vi "Run_Core.vi"(0 "Message Popup in":refnum<class "SMU.lvclass">, 11 "error in (no error)":errorcluster) -> (4 "Message Popup out":refnum<class "SMU.lvclass">, 6 "Return":variant, 15 "error out":errorcluster)   [LabVIEW 2016, in "SMU.lvclass"]
uses:
  SMU.lvclass
  SMU.lvclass/SMU.ctl
  <instrlib>/niDCPower/nidcpower.llb/niDCPower Measurement Type.ctl
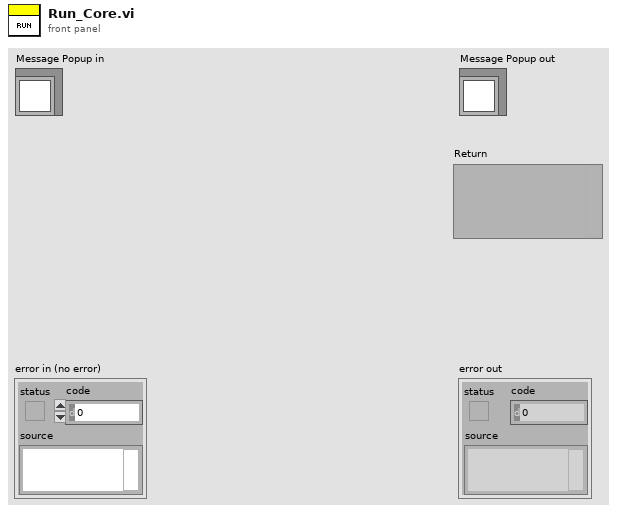
[diagram p1: front panel]
types:
  T1 = typedef "SMU.lvclass/Function List.ctl" = enum16{"init", "source voltage", "source current", "measure voltage", "close", "close all"}
  T2 = typedef "niDCPower Measurement Type.ctl" = i32
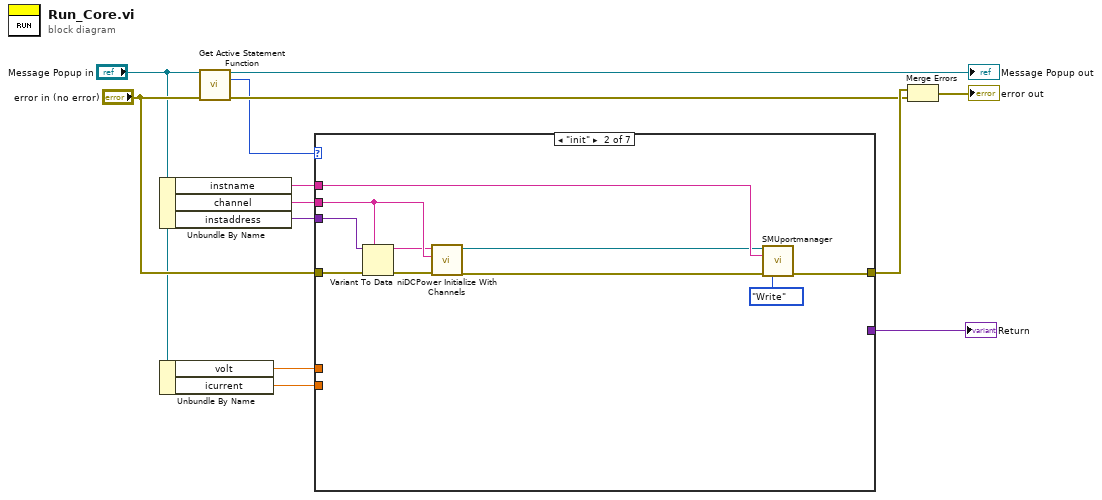
[diagram p0: block diagram]
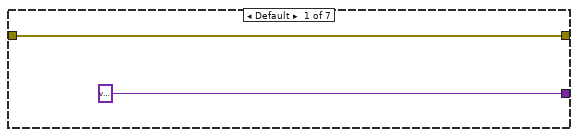
[diagram p2: hidden frame]
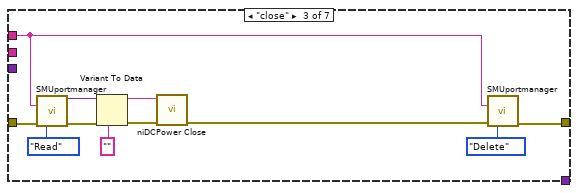
[diagram p3: hidden frame]
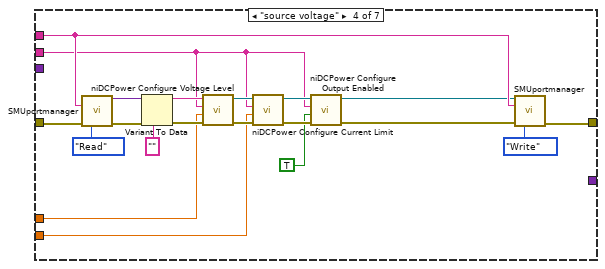
[diagram p4: hidden frame]
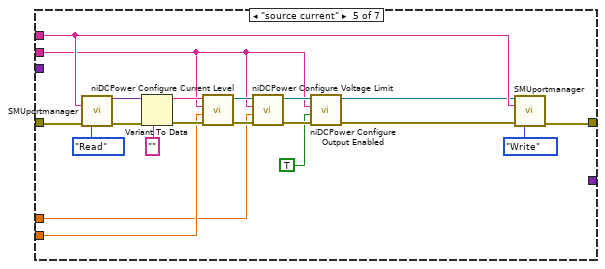
[diagram p5: hidden frame]
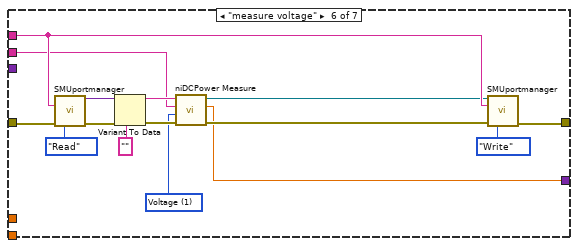
[diagram p6: hidden frame]
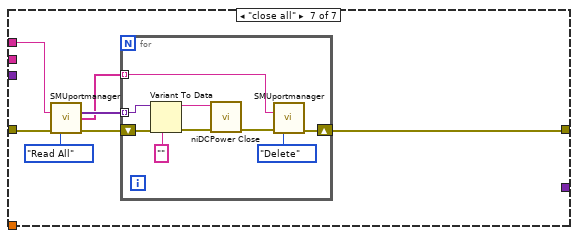
[diagram p7: hidden frame]
diagram:
  n1 = Unbundle By Name("Message Popup in") -> ("instname"=w5:string, "channel"=w4:string, "instaddress"=w11:variant)
  n2 = Unbundle By Name("Message Popup in") -> ("volt"=w2:dbl, "icurrent"=w1:dbl)
  n3 = call "Get Active Statement Function.vi"("Statement in"="Message Popup in", "error in (no error)"="error in (no error)") -> ("Statement out"=→"Message Popup out":refnum<class "SMU.lvclass">, "Function List"=w7:T1, "error out"=w9:errorcluster)  [unwired: 11 in]
  n4 = case shown="\"init\"" w7 {
    tunnel: "error in (no error)" -> [w15 w24 w28 w51 w71 w86 w95]
    tunnel: w11 -> [_ w25 _ _ _ _ _]
    tunnel: [w15 w19 w34 w54 w74 w89 w98] -> w10
    tunnel: [variant ("lefttocomma") _ _ _ _ w77 _] -> w6
    tunnel: w5 -> [_ w22 w27 w50 w70 w85 w94]
    tunnel: w4 -> [_ w17 _ w39 w61 w79 _]
    tunnel: w2 -> [_ _ _ w45 w57 _ _]
    tunnel: w1 -> [_ _ _ w43 w58 _ _]
    frame Default {
    }
    frame "init" {
      n5 = Variant To Data(error in=w24, type=w17, Variant=w25) -> (data=w16:string, error out=w23:errorcluster)
      n6 = call <instrlib>:"niDCPower Initialize With Channels.vi"("error in (no error)"=w23, "channels"=w17, "resource name"=w16) -> ("error out"=w21:errorcluster, "instrument handle out"=w20:refnum<k15>)  [unwired: 7 in]
      n7 = call "SMUportmanager.vi"("port in"=w20, "Name"=w22, "error in (no error)"=w21, "Action"=enum16{"Read", "Write", "Read All", "Delete"}."Write") -> ("error out"=w19:errorcluster)  [unwired: 8 in, 3 out]
    }
    frame "close" {
      n8 = call "SMUportmanager.vi"("Name"=w27, "error in (no error)"=w28, "Action"=enum16{"Read", "Write", "Read All", "Delete"}."Read") -> ("port"=w26:variant, "error out"=w30:errorcluster)  [unwired: 9 in, 2 out]
      n9 = Variant To Data(error in=w30, type="", Variant=w26) -> (data=w33:string, error out=w32:errorcluster)
      n10 = call <instrlib>:"niDCPower Close.vi"("error in (no error)"=w32, "instrument handle"=w33) -> ("error out"=w31:errorcluster)  [unwired: 9 in]
      n11 = call "SMUportmanager.vi"("Name"=w27, "error in (no error)"=w31, "Action"=enum16{"Read", "Write", "Read All", "Delete"}."Delete") -> ("error out"=w34:errorcluster)  [unwired: 9 in, 3 out]
    }
    frame "source voltage" {
      n12 = call "SMUportmanager.vi"("Name"=w50, "error in (no error)"=w51, "Action"=enum16{"Read", "Write", "Read All", "Delete"}."Read") -> ("port"=w49:variant, "error out"=w53:errorcluster)  [unwired: 9 in, 2 out]
      n13 = Variant To Data(error in=w53, type="", Variant=w49) -> (data=w46:string, error out=w48:errorcluster)
      n14 = call <instrlib>:"niDCPower Configure Voltage Level.vi"("error in (no error)"=w48, "voltage level"=w45, "channel name"=w39, "instrument handle"=w46) -> ("error out"=w47:errorcluster, "instrument handle out"=w44:refnum<k15>)  [unwired: 6 in]
      n15 = call <instrlib>:"niDCPower Configure Current Limit.vi"("error in (no error)"=w47, "current limit"=w43, "channel name"=w39, "instrument handle"=w44) -> ("error out"=w41:errorcluster, "instrument handle out"=w42:refnum<k15>)  [unwired: 6 in]
      n16 = call <instrlib>:"niDCPower Configure Output Enabled.vi"("error in (no error)"=w41, "output enabled"=TRUE, "channel name"=w39, "instrument handle"=w42) -> ("error out"=w40:errorcluster, "instrument handle out"=w37:refnum<k15>)  [unwired: 6 in]
      n17 = call "SMUportmanager.vi"("port in"=w37, "Name"=w50, "error in (no error)"=w40, "Action"=enum16{"Read", "Write", "Read All", "Delete"}."Write") -> ("error out"=w54:errorcluster)  [unwired: 8 in, 3 out]
    }
    frame "source current" {
      n18 = call "SMUportmanager.vi"("Name"=w70, "error in (no error)"=w71, "Action"=enum16{"Read", "Write", "Read All", "Delete"}."Read") -> ("port"=w69:variant, "error out"=w73:errorcluster)  [unwired: 9 in, 2 out]
      n19 = Variant To Data(error in=w73, type="", Variant=w69) -> (data=w66:string, error out=w68:errorcluster)
      n20 = call <instrlib>:"niDCPower Configure Current Level.vi"("error in (no error)"=w68, "current level"=w58, "channel name"=w61, "instrument handle"=w66) -> ("error out"=w67:errorcluster, "instrument handle out"=w65:refnum<k15>)  [unwired: 6 in]
      n21 = call <instrlib>:"niDCPower Configure Voltage Limit.vi"("error in (no error)"=w67, "voltage limit"=w57, "channel name"=w61, "instrument handle"=w65) -> ("error out"=w63:errorcluster, "instrument handle out"=w64:refnum<k15>)  [unwired: 6 in]
      n22 = call <instrlib>:"niDCPower Configure Output Enabled.vi"("error in (no error)"=w63, "output enabled"=TRUE, "channel name"=w61, "instrument handle"=w64) -> ("error out"=w62:errorcluster, "instrument handle out"=w59:refnum<k15>)  [unwired: 6 in]
      n23 = call "SMUportmanager.vi"("port in"=w59, "Name"=w70, "error in (no error)"=w62, "Action"=enum16{"Read", "Write", "Read All", "Delete"}."Write") -> ("error out"=w74:errorcluster)  [unwired: 8 in, 3 out]
    }
    frame "measure voltage" {
      w78 = T2 1 items=["Current", "Voltage"] ("measurement type")
      n24 = call "SMUportmanager.vi"("Name"=w85, "error in (no error)"=w86, "Action"=enum16{"Read", "Write", "Read All", "Delete"}."Read") -> ("port"=w84:variant, "error out"=w88:errorcluster)  [unwired: 9 in, 2 out]
      n25 = Variant To Data(error in=w88, type="", Variant=w84) -> (data=w82:string, error out=w83:errorcluster)
      n26 = call <instrlib>:"niDCPower Measure.vi"("error in (no error)"=w83, "measurement type"=w78, "channel name"=w79, "instrument handle"=w82) -> ("error out"=w80:errorcluster, "measurement"=w77:dbl, "instrument handle out"=w81:refnum<k15>)  [unwired: 5 in]
      n27 = call "SMUportmanager.vi"("port in"=w81, "Name"=w85, "error in (no error)"=w80, "Action"=enum16{"Read", "Write", "Read All", "Delete"}."Write") -> ("error out"=w89:errorcluster)  [unwired: 8 in, 3 out]
    }
    frame "close all" {
      n28 = call "SMUportmanager.vi"("Name"=w94, "error in (no error)"=w95, "Action"=enum16{"Read", "Write", "Read All", "Delete"}."Read All") -> ("port[]"=w93:variant[], "port names[]"=w92:string[], "error out"=w97:errorcluster)  [unwired: 9 in, 1 out]
      n29 = for {
        shift-right: [w105] -> w98
        shift-left: w97 -> [w101]
        tunnel: w93 -> [w100] mode=indexing
        tunnel: w92 -> [w99] mode=indexing
        n30 = Variant To Data(error in=w101, type="", Variant=w100) -> (data=w104:string, error out=w103:errorcluster)
        n31 = call <instrlib>:"niDCPower Close.vi"("error in (no error)"=w103, "instrument handle"=w104) -> ("error out"=w102:errorcluster)  [unwired: 9 in]
        n32 = call "SMUportmanager.vi"("Name"=w99, "error in (no error)"=w102, "Action"=enum16{"Read", "Write", "Read All", "Delete"}."Delete") -> ("error out"=w105:errorcluster)  [unwired: 9 in, 3 out]
      }
    }
  }
  "Return" <- w6
  n33 = Merge Errors(w10, w9) -> (→"error out":errorcluster)
